vi "FTW-System-CommandLineToArgv.vi"(0 "Command":string, 11 "error in":errorcluster) -> (6 "**argv":string[](array[string]), 15 "error out":errorcluster)   [LabVIEW 2015]
panel:
  # "Inputs"
  # "Outputs"
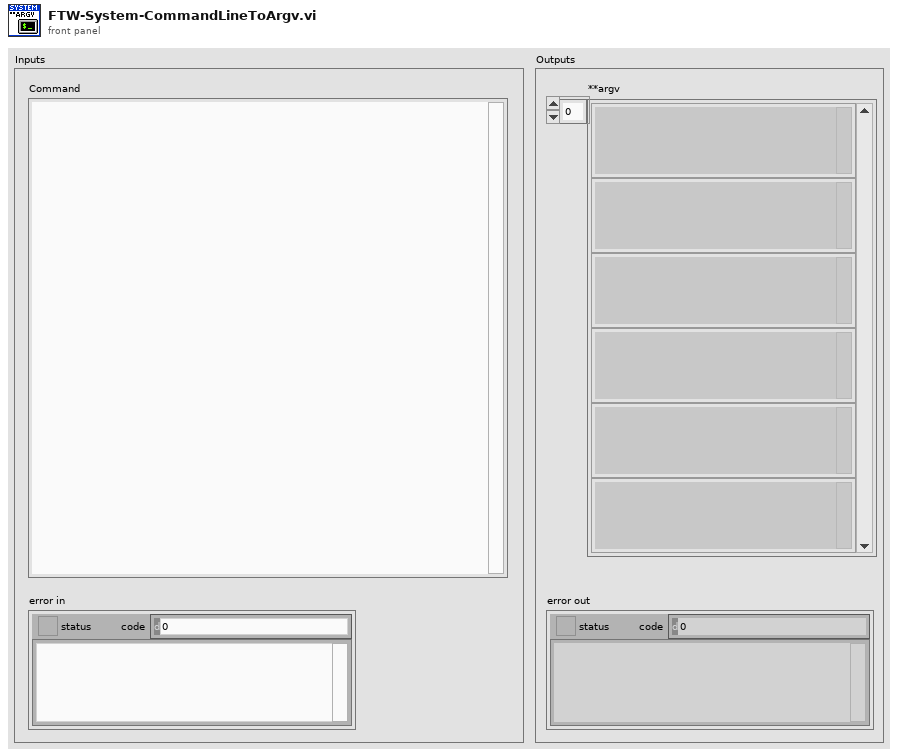
[diagram p1: front panel]
types:
  T1 = typedef "FTW-Type-Regex.ctl" = refnum<data-value>
  T2 = cluster{"callout_id":i32, "subject_current_pos":i32, "subject_start_match_pos":i32, "cap_top":i32, "cap_last":i32, "patt_pos":i32, "callout_name_index":i32, "callout_name_length":i32}[]
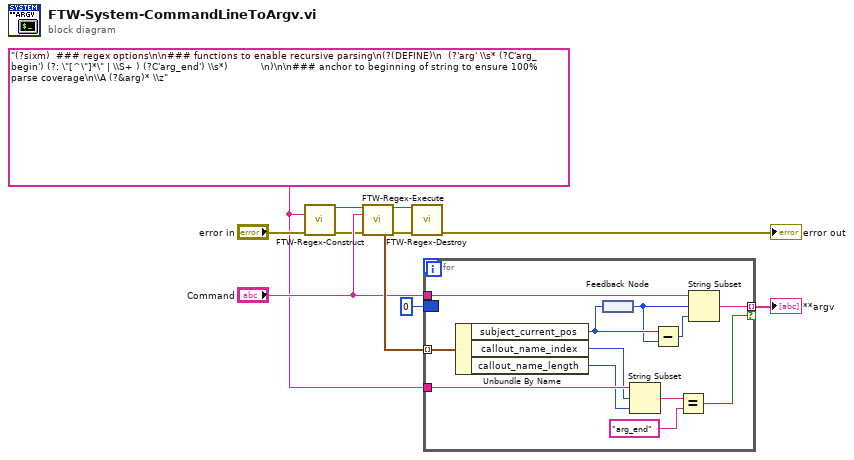
[diagram p0: block diagram]
diagram:
  w3 = "(?sixm)  ### regex options\n\n### functions to enable recursive parsing\n(?(DEFINE)\n  (?'arg' \\s* (?C'arg_begin') (?: \"[^\"]*\" | \\S+ ) (?C'arg_end') \\s*)           \n)\n\n### anchor to beginning of string to ensure 100% parse coverage\n\\A (?&arg)* \\z" ("Regular Expression")
  n1 = call "FTW-Regex-Construct.vi"("Regular Expression"=w3, "error in"="error in") -> ("Regex"=w5:T1, "error out"=w4:errorcluster)  [unwired: 12 in]
  n2 = call "FTW-Regex-Execute.vi"("Regex"=w5, "Subject String"="Command", "error in"=w4) -> ("Regex out"=w11:T1, "Callouts"=w7:T2, "error out"=w8:errorcluster)  [unwired: 7 in, 3 out]
  n3 = call "FTW-Regex-Destroy.vi"("Regex"=w11, "error in"=w8) -> ("error out"=→"error out":errorcluster)  [unwired: 13 in]
  n4 = for {
    tunnel: w7 -> [w23] mode=indexing
    tunnel: "Command" -> [w22]
    tunnel: w3 -> [w20]
    tunnel: [w12] -> w1 mode=indexing if=w15
    border: 0 -> [_]
    n5 = Unbundle By Name(w23) -> ("subject_current_pos"=w14:i32, "callout_name_index"=w19:i32, "callout_name_length"=w18:i32)
    n6 = feedback-in #1(w14) -> ()
    n7 = feedback #1() -> (w13:i32)
    n8 = String Subset(string=w20, offset (0)=w19, length (rest)=w18) -> (substring=w17:string)
    n9 = Subtract(x=w14, y=w13) -> (x-y=w21:i32)
    n10 = Equal?(x=w17, y="arg_end") -> (x = y?=w15:bool)
    n11 = String Subset(string=w22, offset (0)=w13, length (rest)=w21) -> (substring=w12:string)
  }
  "**argv" <- w1
